vi "Node ID.vi"(11 "Module in":refnum<class "Module.lvclass">) -> (2 "Node ID":u32, 3 "Module out":refnum<class "Module.lvclass">)   [LabVIEW 2020, in "Volatus.lvlib" / "Module.lvclass"]
uses:
  Module.lvclass
  Module.lvclass/Module.ctl
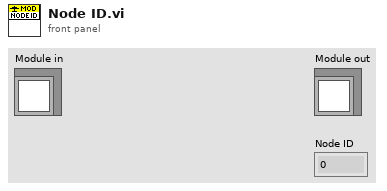
[diagram p1: front panel]
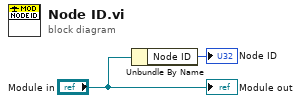
[diagram p0: block diagram]
diagram:
  n1 = Unbundle By Name("Module in") -> ("Node ID"=→"Node ID":u32)
  "Module out" <- "Module in"
